vi "Process File.vi"(8 "error in (no error)":errorcluster, 10 "Result in":refnum<class "Acquired Result.lvclass">, 11 "Elastic Moduli in":refnum<class "Elastic Moduli.lvclass">) -> (0 "error out":errorcluster, 2 "Result out":refnum<class "Acquired Result.lvclass">, 3 "Elastic Moduli out":refnum<class "Elastic Moduli.lvclass">)   [LabVIEW 2016, in "Elastic Moduli.lvclass"]
uses:
  Elastic Moduli.lvclass
  C:/github/LabActor/Worker/Worker.lvclass
  NHMFL_Core/Libraries/Instruments/Results/Acquired Result/Acquired Result.lvclass
  Worker/Worker.lvclass/Worker.ctl
  Worker/Read File Path.vi
  <vilib>/express/express shared/transition.llb/Dynamic To Waveform Array.vi
  Read Elastic Moduli Configuration.vi
  <vilib>/express/express signal manip/GetorSetDDTAttributes/Get DDT Attributes/Get DDT Properties.xnode
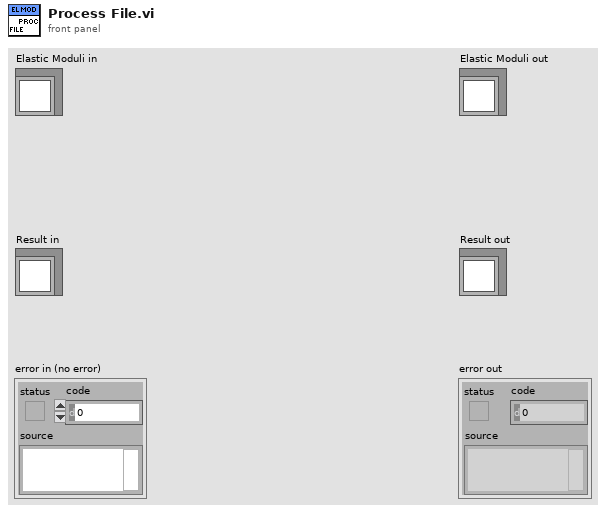
[diagram p1: front panel]
types:
  T1 = typedef "Elastic Moduli Configuration.ctl" = cluster{"Output header ":string, "rusin\n.dat":enum16{"NONE", "DINES/cm2", "GPa"}, "Line detector module name":string, "Modulas output file":path}
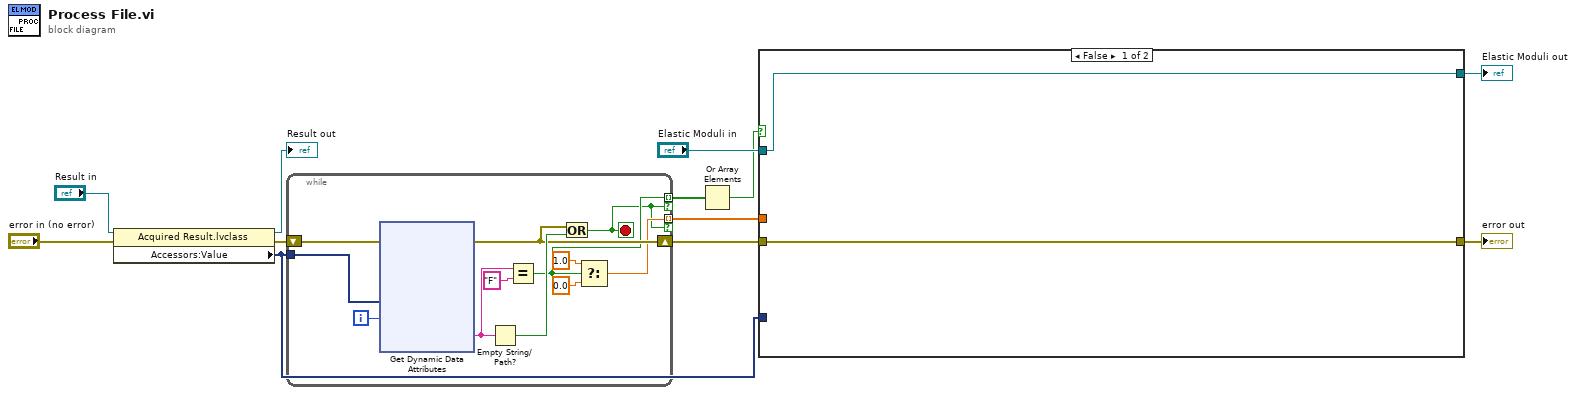
[diagram p0: block diagram]
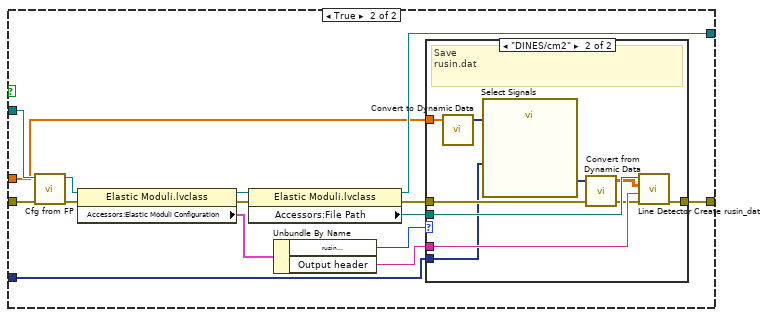
[diagram p2: hidden frame]
diagram:
  n1 = property class="Acquired Result.lvclass"(reference="Result in", error in="error in (no error)") -> (reference out=→"Result out":refnum<class "Acquired Result.lvclass">, error out=w2:errorcluster, "Accessors:Value"=w8:dynamicdata)
  n2 = while {
    tunnel: w8 -> [w24]
    shift-right: [w19] -> w3
    shift-left: w2 -> [w20]
    tunnel: [w17] -> w5 mode=indexing if=w13
    tunnel: [w14] -> w7 mode=indexing if=w13
    i -> [w18]
    stop <- w13 stop-if-true
    n3 = xnode "Get Dynamic Data Attributes"("Signals In"=w24, "Signal Index"=w18, "error in"=w20) -> ("Signal Name"=w21:string, "error out"=w19:errorcluster)  [unwired: 1 out]
    n4 = Empty String/Path?(string/path=w21) -> (empty?=w22:bool)
    n5 = Equal?(x=w21, y="F" ("Signal Name")) -> (x = y?=w17:bool)
    n6 = Or(x=w19, y=w22) -> (x .or. y?=w13:bool)
    n7 = Select(t=1.0, s=w17, f=0.0) -> (s? t:f=w14:dbl)
  }
  n8 = Or Array Elements(Boolean array=w5) -> (logical OR=w4:bool)
  n9 = case shown="False" w4 {
    tunnel: "Elastic Moduli in" -> [w35 w48]
    tunnel: [w35 w41] -> w11
    tunnel: [w34 w39] -> w10
    tunnel: w8 -> [_ w38]
    tunnel: w7 -> [_ w37]
    tunnel: w3 -> [w34 w36]
    frame False {
    }
    frame True {
      n10 = call-dynamic "Cfg from FP.vi"("error in (no error)"=w36, "Measure Object in"=w48) -> ("error out"=w43:errorcluster, "Measure Object out"=w49:refnum<class "Elastic Moduli.lvclass">)  [unwired: 8 in]
      n11 = property class="Elastic Moduli.lvclass"(reference=w49, error in=w43) -> (reference out=w42:refnum<class "Elastic Moduli.lvclass">, error out=w50:errorcluster, "Accessors:Elastic Moduli Configuration"=w47:T1)
      n12 = property class="Elastic Moduli.lvclass"(reference=w42, error in=w50) -> (reference out=w41:refnum<class "Elastic Moduli.lvclass">, error out=w40:errorcluster, "Accessors:File Path"=w45:path)
      n13 = Unbundle By Name(w47) -> ("rusin\n.dat"=w46:enum16{"NONE", "DINES/cm2", "GPa"}, "Output header"=w44:string)
      n14 = case shown="\"DINES/cm2\"" w46 {
        tunnel: w44 -> [_ w59]
        tunnel: w45 -> [_ w60]
        tunnel: w40 -> [w51 w58]
        tunnel: [w51 w57] -> w39
        tunnel: w38 -> [_ w56]
        tunnel: w37 -> [_ w55]
        frame "NONE", Default {
        }
        frame "DINES/cm2" {
          # "Save\nrusin.dat"
          n15 = call "Convert to Dynamic Data"("Array"=w55) -> ("Dynamic Data Type"=w54:dynamicdata)  [unwired: 3 in]
          n16 = call "Select Signals"("Selector Input"=w54, "Signals"=w56) -> ("Signal Out"=w53:dynamicdata)  [unwired: 8 in, 1 out]
          n17 = call "Convert from Dynamic Data"("Dynamic Data Type"=w53) -> ("Array"=w52:dbl[][])  [unwired: 3 in]
          n18 = call "Line Detector Create rusin_dat.vi"("Error In"=w58, "header"=w59, "Fit results"=w52, "File Path Control"=w60) -> ("Error Out"=w57:errorcluster)  [unwired: 7 in]
        }
      }
    }
  }
  "error out" <- w10
  "Elastic Moduli out" <- w11
